vi "Obtain DAQ Experimental Queue.vi"() -> (0 "Experimental DAQ Queue":T1)   [LabVIEW 2013]
uses:
  Runtime Queue.ctl
  Experimental Configuration.ctl
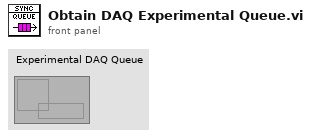
[diagram p1: front panel]
types:
  T1 = typedef "Runtime Queue.ctl" = refnum<queue>
  T2 = typedef "Experimental Configuration.ctl" = cluster{"Output Waveforms":waveform(dbl)[], "Output Channels":string, "Input Channels":string, "Post-Hook Occurence":refnum<k4>}
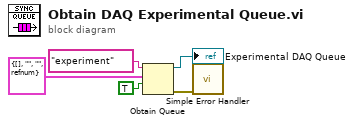
[diagram p0: block diagram]
diagram:
  n1 = Obtain Queue(name (unnamed)="experiment", element data type=T2 {"Output Waveforms"=[], "Output Channels"="", "Input Channels"="", "Post-Hook Occurence"=refnum} ("Experimental Configuration"), create if not found? (T)=TRUE) -> (queue out=→"Experimental DAQ Queue":refnum<queue>, error out=w2:errorcluster)  [unwired: 2 in, 1 out]
  n2 = call <vilib>:"Simple Error Handler.vi"("error in (no error)"=w2) -> ()  [unwired: 4 in, 5 out]
